vi "save_vi.vi"(8 "error in (no error)":errorcluster, 10 "VI Path":path, 11 "vi reference":refnum<vi>) -> (0 "error out":errorcluster, 3 "vi reference out":refnum<vi>)   [LabVIEW 2018]
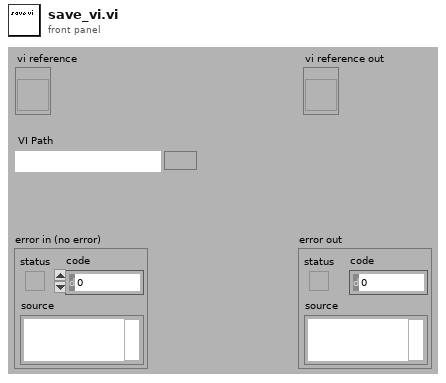
[diagram p1: front panel]
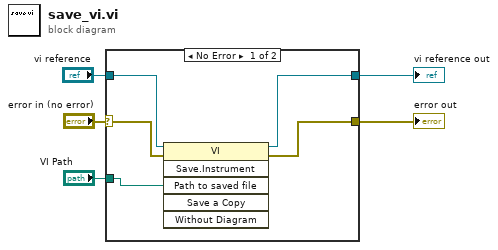
[diagram p0: block diagram]
diagram:
  n1 = case shown="No Error" "error in (no error)" {
    selector: "error in (no error)" -> [w9 w12]
    tunnel: [w7 w12] -> w3
    tunnel: "vi reference" -> [w10 w11]
    tunnel: [w8 w11] -> w2
    tunnel: "VI Path" -> [w6 _]
    frame No Error {
      n2 = invoke class="VI" method="Save.Instrument"(reference=w10, error in=w9, "Path to saved file"=w6) -> (reference out=w8:refnum<vi>, error out=w7:errorcluster)  [unwired: 3 in, 4 out]
    }
    frame Error {
    }
  }
  "error out" <- w3
  "vi reference out" <- w2
